vi "解析波特率.vi"(1 "GPRS参数":i32) -> (0 "波特率":i32)   [LabVIEW 2015]
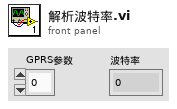
[diagram p1: front panel]
types:
  T1 = typedef "GPRS波特率参数.ctl" = i32[]
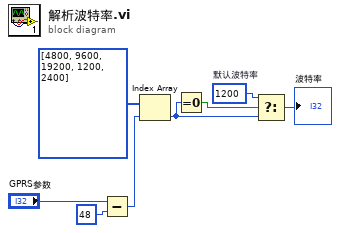
[diagram p0: block diagram]
diagram:
  w2 = 1200  # 默认波特率
  n1 = Subtract(x="GPRS参数", y=u16 48) -> (x-y=w6:i32)
  n2 = Index Array(array=T1 [4800, 9600, 19200, 1200, 2400] ("数组"), index=w6) -> (element=w1:i32)
  n3 = Equal To 0?(x=w1) -> (x = 0?=w4:bool)
  n4 = Select(t=w2, s=w4, f=w1) -> (s? t:f=→"波特率":i32)
